vi "Calc X & Y Desired Velocity.vi"(8 "x goal":dbl, 9 "x start":dbl, 10 "Y Goal":dbl, 11 "Y Position":dbl) -> (0 "robot desired velocity x component\n u1 (ft/s)":dbl, 3 "robot desired velocity y component\n u2 (ft/s)":dbl)   [LabVIEW 2015]
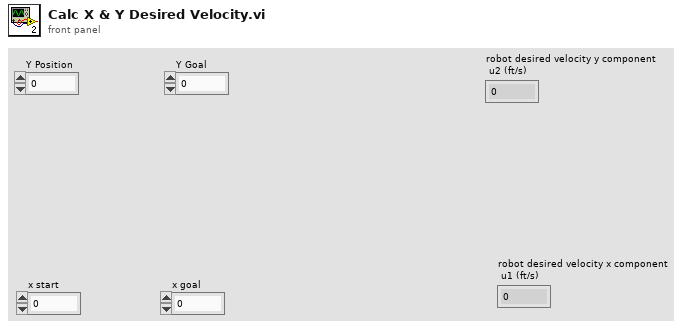
[diagram p1: front panel]
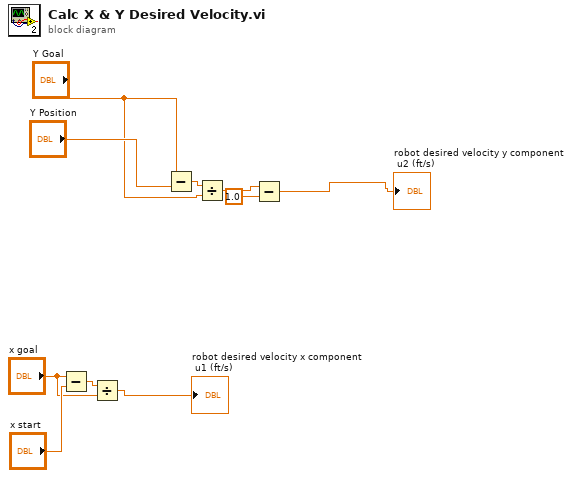
[diagram p0: block diagram]
diagram:
  n1 = Subtract(x="x goal", y="x start") -> (x-y=w7:dbl)
  n2 = Divide(x=w7, y="x goal") -> (x/y=→"robot desired velocity x component\n u1 (ft/s)":dbl)
  n3 = Subtract(x="Y Goal", y="Y Position") -> (x-y=w10:dbl)
  n4 = Divide(x=w10, y="Y Goal") -> (x/y=w3:dbl)
  n5 = Subtract(x=w3, y=1.0) -> (x-y=→"robot desired velocity y component\n u2 (ft/s)":dbl)
